vi "test Send Message.vi"(8 "error in (no error)":errorcluster, 11 "TestCase in":refnum<class "Test TCP Stream Transmission.lvclass">) -> (0 "error out":errorcluster, 3 "TestCase out":refnum<class "Test TCP Stream Transmission.lvclass">)   [LabVIEW 2020, in "Test TCP Stream Transmission.lvclass"]
uses:
  Test TCP Stream Transmission.lvclass
  <vilib>/ActorFramework/LastAck/Last Ack.lvclass
  <vilib>/ActorFramework/Message/Message.lvclass
  <vilib>/addons/_JKI Toolkits/VI Tester/TestCase.llb/TestCase.lvclass
  Source/Protocols/TCP Strategy/TCP Stream Initiator/TCP Stream Initiator.lvclass
  Source/Abstract Classes/Cipher/Cipher.lvclass
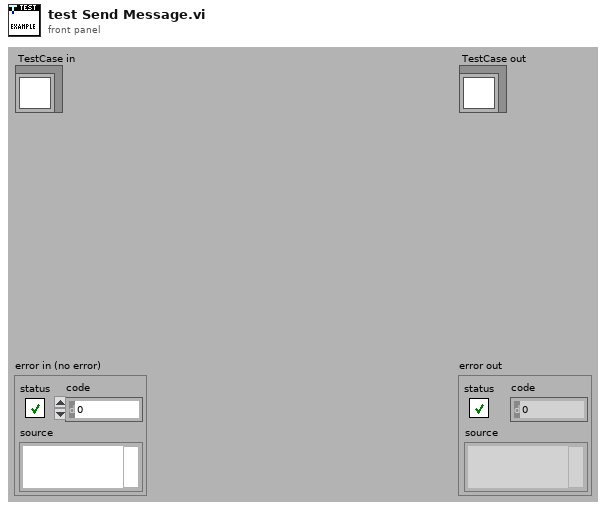
[diagram p1: front panel]
types:
  T1 = enum16{"Standard", "Buffered", "CRLF", "Immediate"}
  T2 = cluster{"Actor Framework:Message":refnum<class "Message.lvclass">, "priority":i32}
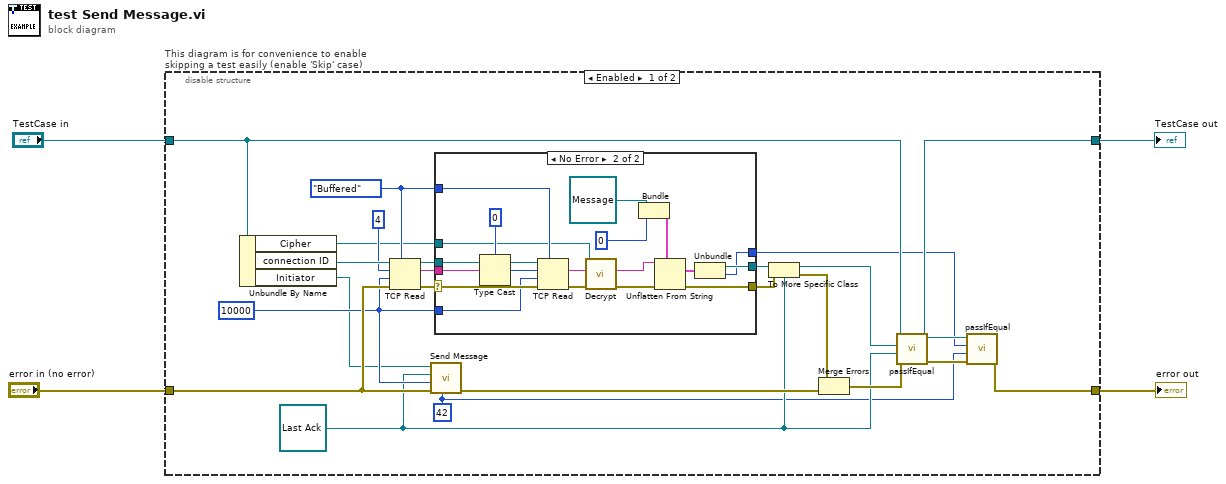
[diagram p0: block diagram]
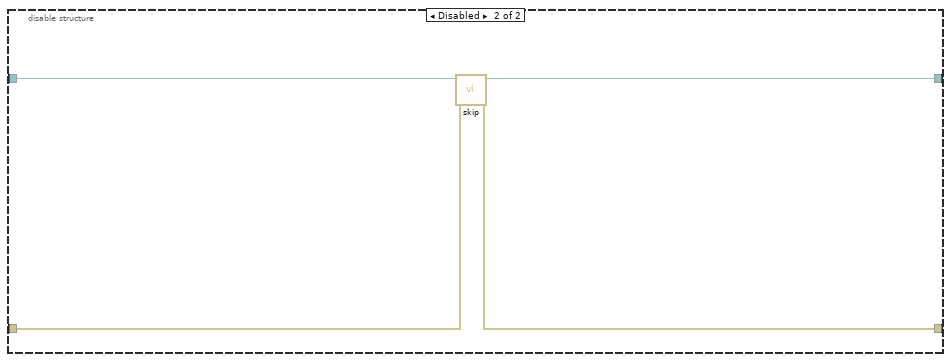
[diagram p3: hidden frame]
diagram:
  n1 = disable-structure "This diagram is for convenience to enable skipping a test easily (enable 'Skip' case)" shown="Enabled" {
    disable-tunnel: "TestCase in" -> [w21 w51]
    disable-tunnel: [w10 w49] -> w3
    disable-tunnel: [w7 w50] -> w2
    disable-tunnel: "error in (no error)" -> [w19 w48]
    frame Enabled {
      w8 = 42 ("priority")
      w12 = refnum<class "Last Ack.lvclass"> refnum ("Last Ack")
      w18 = 10000 ("timeout ms (25000)")
      w27 = T1."Buffered" ("mode (standard)")
      n2 = Unbundle By Name(w21) -> ("Cipher"=w5:refnum<class "Cipher.lvclass">, "connection ID"=w26:refnum<k5>, "Initiator"=w17:refnum<class "TCP Stream Initiator.lvclass">)
      n3 = TCP Read(connection ID=w26, bytes to read=4, error in (no error)=w19, 7:w27, 9:w18) -> (connection ID out=w24:refnum<k5>, data out=w23:string, error out=w25:errorcluster)
      n4 = call-dynamic "Send Message.vi"("priority"=w8, "error in (no error)"=w19, "timeout ms (-1)"=w18, "Message"=w12, "TCP Stream in"=w17) -> ("error out"=w20:errorcluster)  [unwired: 5 in, 1 out]
      n5 = case shown="No Error" w25 {
        selector: w25 -> [w28 w43]
        tunnel: w23 -> [_ w47]
        tunnel: [w28 w40] -> w15
        tunnel: w24 -> [_ w44]
        tunnel: w18 -> [_ w42]
        tunnel: w27 -> [_ w41]
        tunnel: [_ w35] -> w16
        tunnel: [_ w34] -> w6
        tunnel: w5 -> [_ w29]
        frame Error {
        }
        frame No Error {
          n6 = Type Cast(type=0 ("bytes to read"), x=w47) -> (*(type *) &x=w45:i32)
          n7 = TCP Read(connection ID=w44, bytes to read=w45, error in (no error)=w43, 7:w41, 9:w42) -> (data out=w31:string, error out=w33:errorcluster)  [unwired: 1 out]
          n8 = call-dynamic "Decrypt.vi"("error in (no error)"=w33, "Ciphertext"=w31, "Cipher in"=w29) -> ("error out"=w32:errorcluster, "Plaintext"=w30:string)  [unwired: 6 in, 1 out]
          n9 = Bundle("Actor Framework:Message"=refnum<class "Message.lvclass"> refnum, "priority"=0) -> (w37:T2)  [unwired: 1 in]
          n10 = Unflatten From String(type=w37, binary string=w30, error in (no error)=w32) -> (value=w36:T2, error out=w40:errorcluster)  [unwired: 2 in, 1 out]
          n11 = Unbundle(w36) -> ("Actor Framework:Message"=w35:refnum<class "Message.lvclass">, "priority"=w34:i32)
        }
      }
      n12 = To More Specific Class(target class=w12, reference=w16, error in=w15) -> (specific class reference=w11:refnum<class "Last Ack.lvclass">, error out=w13:errorcluster)
      n13 = Merge Errors(w13, w20) -> (w14:errorcluster)
      n14 = call-dynamic "passIfEqual.vi"("error in (no error)"=w14, "y"=w12, "x"=w11, "TestCase in"=w21) -> ("error out"=w9:errorcluster, "TestCase out"=w10:refnum<class "Test TCP Stream Transmission.lvclass">)  [unwired: 6 in]
      n15 = call-dynamic "passIfEqual.vi"("error in (no error)"=w9, "y"=w8, "x"=w6, "TestCase in"=w10) -> ("error out"=w7:errorcluster)  [unwired: 6 in, 1 out]
    }
    frame Disabled {
      # "skip test result while test is under development"
      n16 = call <vilib>:"skip.vi"("error in (no error)"=w48, "TestCase in"=w51) -> ("error out"=w50:errorcluster, "TestCase out"=w49:refnum<class "Test TCP Stream Transmission.lvclass">)  [unwired: 8 in]
    }
  }
  "error out" <- w2
  "TestCase out" <- w3
